vi "OCV Measure.vi"(8 "error in (no error)":errorcluster, 11 "Refnum in":refnum<k21>) -> (0 "error out":errorcluster, 1 "Voltage":sgl[](array[numeric])=[3.481668, 3.483052, 3.4783623, 3.4823976, 3.484474] format="%#_8g", 3 "Refnum out":refnum<k21>, 4 "Read Time (ms)":u32=46)   [LabVIEW 2019]
uses:
  <vilib>/DAQmx/miscellaneous.llb/DAQmx Fill In Error Info.vi
  <vilib>/DAQmx/read.llb/DAQmx Read (Analog 1D DBL NChan 1Samp).vi
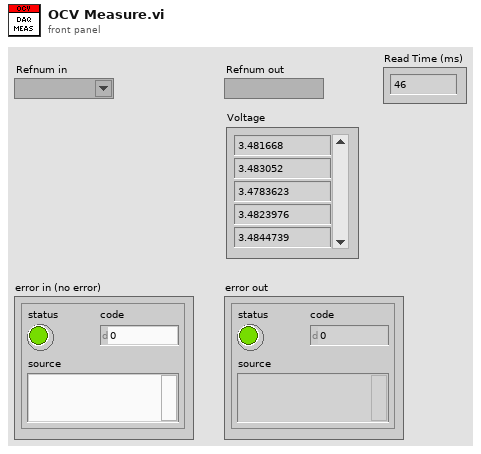
[diagram p1: front panel]
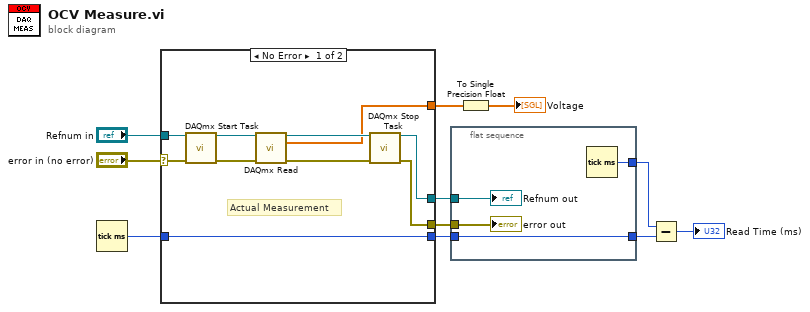
[diagram p0: block diagram]
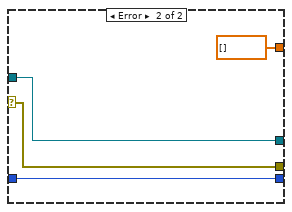
[diagram p2: hidden frame]
diagram:
  n1 = Tick Count (ms)() -> (millisecond timer value=w4:u32)
  n2 = case shown="No Error" "error in (no error)" {
    selector: "error in (no error)" -> [w14 w24]
    tunnel: [w12 sgl[] []] -> w1
    tunnel: "Refnum in" -> [w17 w25]
    tunnel: [w16 w25] -> w7
    tunnel: [w15 w24] -> w6
    tunnel: w4 -> [w13 w23]
    tunnel: [w13 w23] -> w3
    frame No Error {
      # "Actual Measurement"
      n3 = call <vilib>:"DAQmx Start Task.vi"("task/channels in"=w17, "error in"=w14) -> ("task out"=w20:refnum<k21>, "error out"=w21:errorcluster)  [unwired: 12 in]
      n4 = call-poly <vilib>:"DAQmx Read.vi"("task/channels in"=w20, "error in"=w21) -> ("task out"=w19:refnum<k21>, "data"=w12:dbl[], "error out"=w18:errorcluster)  [unwired: 11 in]
      n5 = call <vilib>:"DAQmx Stop Task.vi"("task/channels in"=w19, "error in"=w18) -> ("task out"=w16:refnum<k21>, "error out"=w15:errorcluster)  [unwired: 12 in]
    }
    frame Error {
    }
  }
  n6 = flat-sequence {
    tunnel: [w29] -> w8
    tunnel: w3 -> [w28]
    tunnel: [w28] -> w9
    tunnel: w7 -> [w27]
    tunnel: w6 -> [w26]
    frame #0 {
      n7 = Tick Count (ms)() -> (millisecond timer value=w29:u32)
      "Refnum out" <- w27
      "error out" <- w26
    }
  }
  n8 = To Single Precision Float(number=w1) -> (single precision float=→"Voltage":sgl[])
  n9 = Subtract(x=w8, y=w9) -> (x-y=→"Read Time (ms)":u32)
